vi "csmdoc_import_VI_description.vi"(8 "error in (no error)":errorcluster, 9 "NOTE-Map":variant, 10 "string":string, 11 "Path":path) -> (0 "error out":errorcluster)   [LabVIEW 2017, in "csmdoc.lvlib"]
uses:
  csmdoc.lvlib
  Communicable State Machine.lvlib
panel:
  out "Array 2":bool[](array[boolean])
  out "Variant":variant
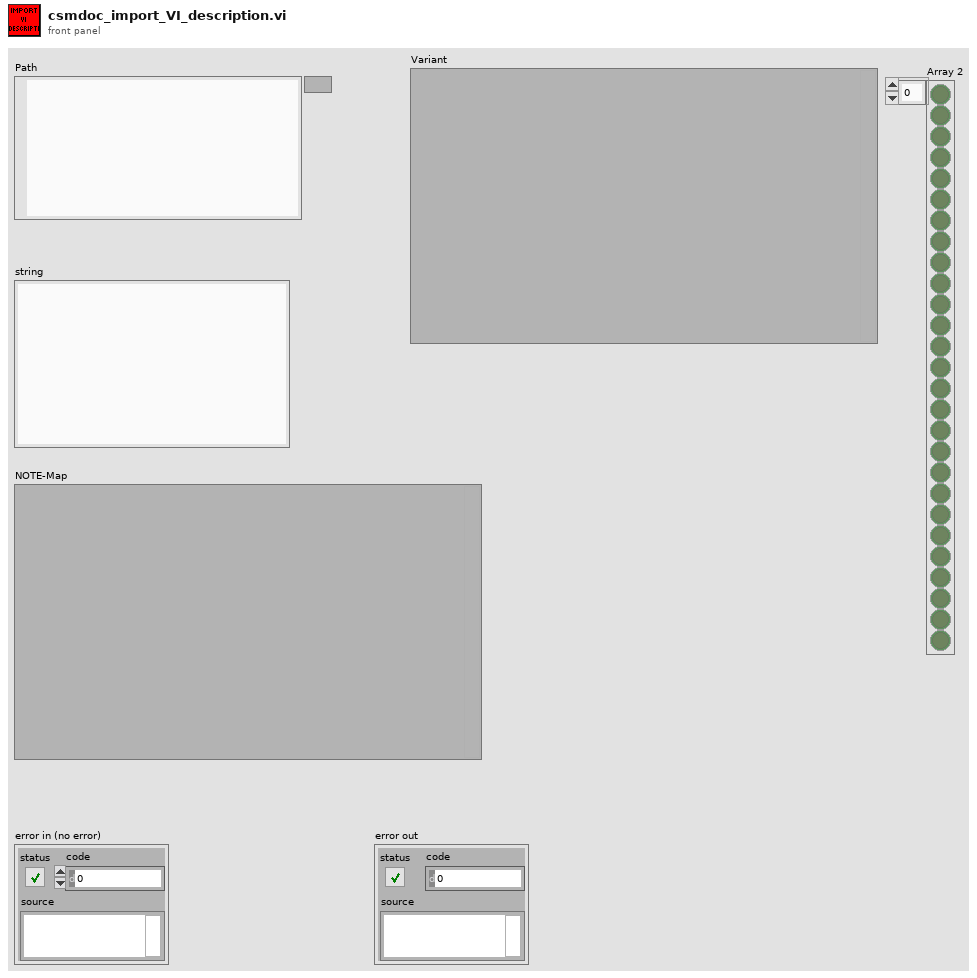
[diagram p1: front panel]
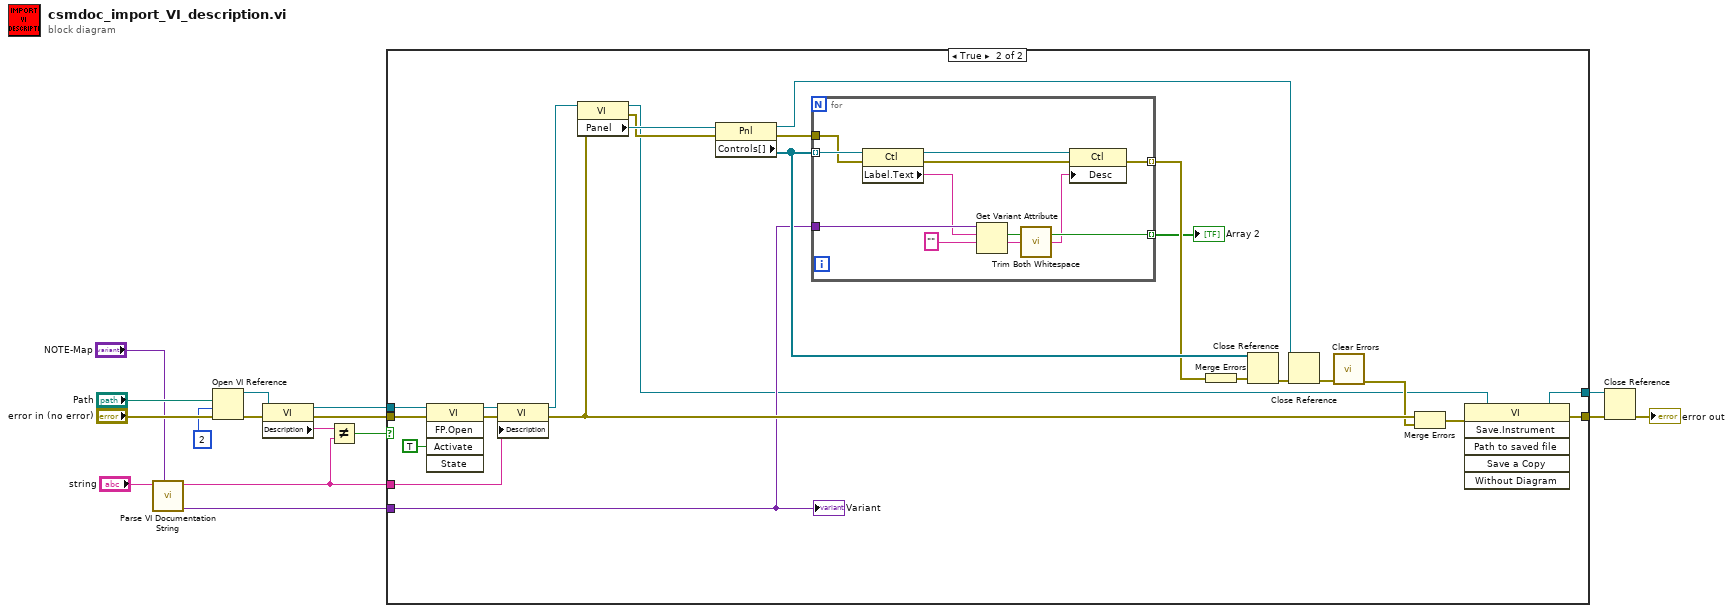
[diagram p0: block diagram]
diagram:
  n1 = call "Parse VI Documentation String.vi"("NOTE-Map"="NOTE-Map", "Documentation"="string") -> ("Ctrl-Doc Map"=w10:variant, "Documentation (dup)"=w4:string)  [unwired: 6 in, 2 out]
  n2 = Open VI Reference(vi path="Path", options=2, error in (no error)="error in (no error)") -> (vi reference=w9:refnum<vi>, error out=w16:errorcluster)  [unwired: 3 in]
  n3 = property class="VI"(reference=w9, error in=w16) -> (reference out=w6:refnum<vi>, error out=w7:errorcluster, "Description"=w5:string)
  n4 = Not Equal?(x=w5, y=w4) -> (x != y?=w1:bool)
  n5 = case shown="True" w1 {
    tunnel: w10 -> [_ w29]
    tunnel: w7 -> [w18 w20]
    tunnel: w6 -> [w17 w19]
    tunnel: w4 -> [_ w28]
    tunnel: [w18 w26] -> w3
    tunnel: [w17 w24] -> w2
    frame False {
    }
    frame True {
      n6 = invoke class="VI" method="FP.Open"(reference=w19, error in=w20, "Activate"=TRUE ("Activate?")) -> (reference out=w22:refnum<vi>, error out=w21:errorcluster)  [unwired: 2 in, 3 out]
      n7 = property class="VI"(reference=w22, error in=w21, "Description"=w28) -> (reference out=w42:refnum<vi>, error out=w33:errorcluster)
      n8 = property class="VI"(reference=w42, error in=w33) -> (reference out=w25:refnum<vi>, error out=w40:errorcluster, "Panel"=w41:refnum<vi>)
      n9 = property class="Pnl"(reference=w41, error in=w40) -> (reference out=w34:refnum<vi>, error out=w37:errorcluster, "Controls[]"=w39:refnum<vi>[])
      n10 = for {
        tunnel: w39 -> [w53] mode=indexing
        tunnel: w37 -> [w52]
        tunnel: [w49] -> w36 mode=indexing
        tunnel: w29 -> [w48]
        tunnel: [w44] -> w30 mode=indexing
        n11 = property class="Ctl"(reference=w53, error in=w52) -> (reference out=w51:refnum<vi>, error out=w50:errorcluster, "Label.Text"=w47:string)
        n12 = Get Variant Attribute(Variant=w48, name=w47, default value (empty Variant)="" ("regular expression")) -> (found=w44:bool, value=w45:string)  [unwired: 1 in, 2 out]
        n13 = call "Trim Both Whitespace.vi"("string"=w45) -> ("trimmed string"=w43:string)  [unwired: 1 in]
        n14 = property class="Ctl"(reference=w51, error in=w50, "Desc"=w43) -> (error out=w49:errorcluster)  [unwired: 1 out]
      }
      "Array 2" <- w30
      n15 = Merge Errors(w36) -> (w35:errorcluster)
      n16 = Close Reference(reference=w39, error in (no error)=w35) -> (error out=w38:errorcluster)
      n17 = Close Reference(reference=w34, error in (no error)=w38) -> (error out=w32:errorcluster)
      n18 = call <vilib>:"Clear Errors.vi"("error in (no error)"=w32) -> ("error out"=w31:errorcluster)  [unwired: 5 in, 1 out]
      n19 = Merge Errors(w33, w31) -> (w27:errorcluster)
      n20 = invoke class="VI" method="Save.Instrument"(reference=w25, error in=w27) -> (reference out=w24:refnum<vi>, error out=w26:errorcluster)  [unwired: 4 in, 4 out]
      "Variant" <- w29
    }
  }
  n21 = Close Reference(reference=w2, error in (no error)=w3) -> (error out=→"error out":errorcluster)
